vi "Read Read Only.vi"(8 "error in (no error)":errorcluster, 11 "Const_U64 in":refnum<class "Const_U64.lvclass">) -> (0 "error out":errorcluster, 2 "Read Only":bool, 3 "Const_U64 out":refnum<class "Const_U64.lvclass">)   [LabVIEW 2021, in "Const_U64.lvclass"]
uses:
  Const_U64.lvclass
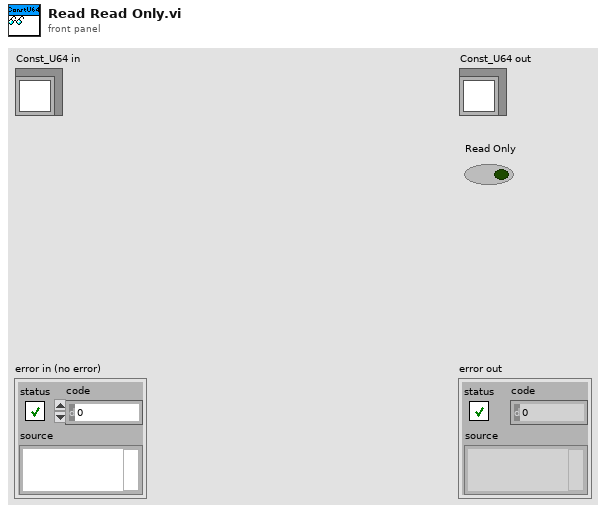
[diagram p1: front panel]
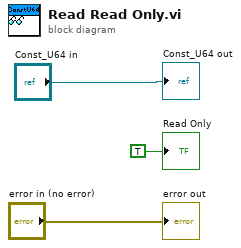
[diagram p0: block diagram]
diagram:
  "error out" <- "error in (no error)"
  "Const_U64 out" <- "Const_U64 in"
  "Read Only" <- TRUE ("Read Only")
